vi "Neurosky.vi"() -> ()   [LabVIEW 2011]
uses:
  <vilib>/measure/maspectr.llb/FFT Power Spectrum and PSD for 1 Chan.vi
  Neurosky.lvlib
  <vilib>/measure/NI_MAPro.lvlib
panel:
  out "Mindwave Braiwave Data":T1
  out "FFT Power Spectrum":cluster{"f0":dbl, "df":dbl, "magnitude":dbl[]}(graph)
  out "Mindwave Common Signals\nMobile Data":T2 {"Meditation" scale=0.0..100.0; "Attention" scale=0.0..100.0; "Poor Signal Strength" scale=0.0..255.0}
  out "RAW Wave":waveform(i16)(graph)
  in  "Baud Rate":u16(ring)=10 items=["300", "600", "900", "1200", "2400", "4800", "9600", "19200", "38400", "57600", "115200", "230400"]
  in  "Comm Port":refnum<visa-resource-name>="COM4"
  in  "Start Button":bool
  in  "Stop Button":bool
  # "Visit http://www.cerescontrols.com"
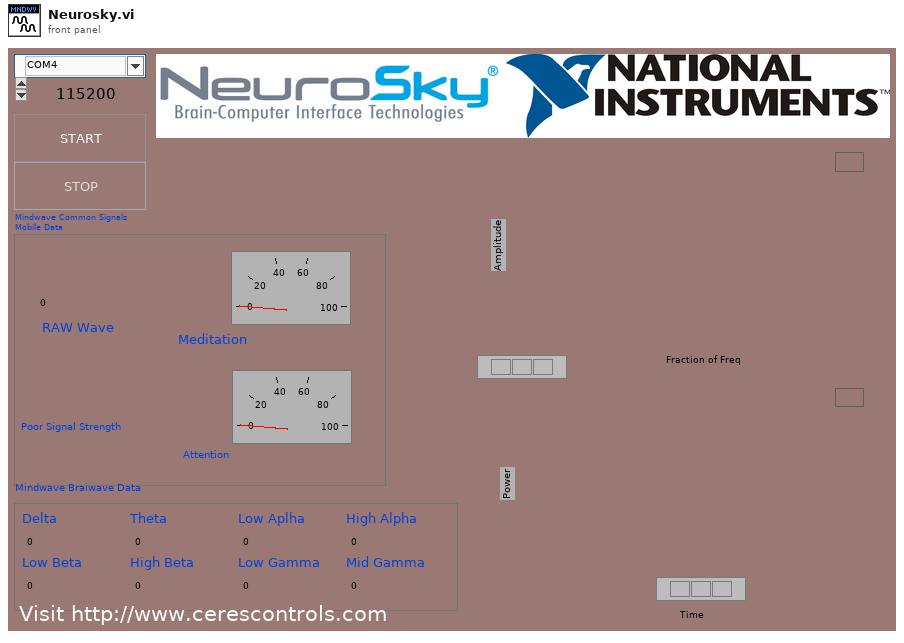
[diagram p1: front panel]
types:
  T1 = cluster{"Delta":sgl, "Theta":sgl, "Low Aplha":sgl, "High Alpha":sgl, "Low Beta":sgl, "High Beta":sgl, "Low Gamma":sgl, "Mid Gamma":sgl}
  T2 = cluster{"RAW Wave":i16, "Poor Signal Strength":u8, "Attention":u16, "Meditation":u8}
  T3 = enum8{"Enabled", "Disabled", "Disabled and Grayed Out"}
  T4 = cluster{"RAW_WAVE":i16, "POOR_QUALITY":u8, "delta":sgl, "theta":sgl, "low alpha":sgl, "high alpha":sgl, "low beta":sgl, "high beta":sgl, "low gamma":sgl, "mid gamma":sgl, "ATTENTION":u8, "MEDITATION":u8}
  T5 = cluster{"delta":sgl, "theta":sgl, "low alpha":sgl, "high alpha":sgl, "low beta":sgl, "high beta":sgl, "low gamma":sgl, "mid gamma":sgl}
  T6 = cluster{"RAW_WAVE":i16, "POOR_QUALITY":u8, "ATTENTION":u8, "MEDITATION":u8}
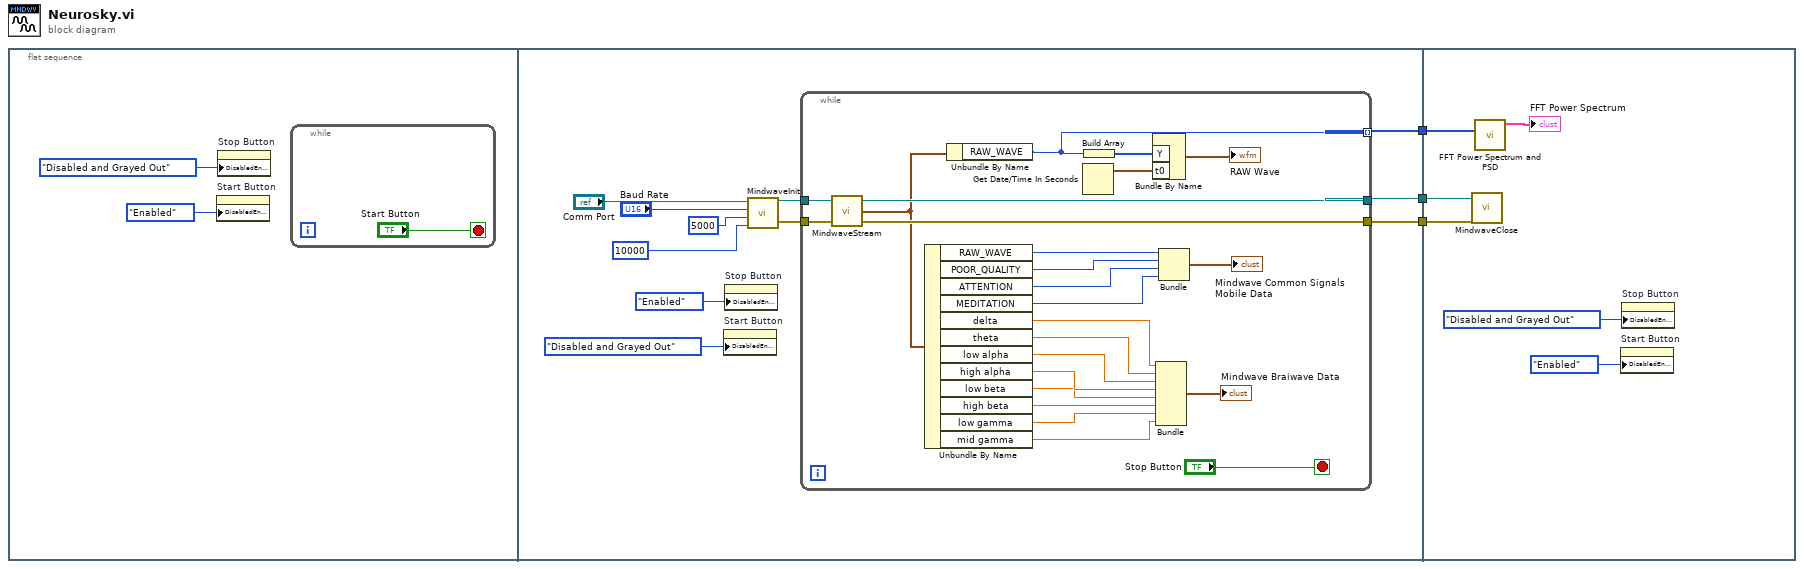
[diagram p0: block diagram]
diagram:
  n1 = flat-sequence {
    tunnel: [w11] -> w3
    tunnel: [w10] -> w2
    tunnel: [w9] -> w1
    tunnel: w3 -> [w47]
    tunnel: w2 -> [w46]
    tunnel: w1 -> [w45]
    frame #0 {
      n2 = property on="Start Button" class="Bool"("DisabledEnum"=T3."Enabled" ("Disabled")) -> ()  [unwired: 2 in, 2 out]
      n3 = property on="Stop Button" class="Bool"("DisabledEnum"=T3."Disabled and Grayed Out" ("Disabled")) -> ()  [unwired: 2 in, 2 out]
      n4 = while {
        stop <- "Start Button" stop-if-true
      }
    }
    frame #1 {
      n5 = property on="Start Button" class="Bool"("DisabledEnum"=T3."Disabled and Grayed Out" ("Disabled")) -> ()  [unwired: 2 in, 2 out]
      n6 = property on="Stop Button" class="Bool"("DisabledEnum"=T3."Enabled" ("Disabled")) -> ()  [unwired: 2 in, 2 out]
      n7 = call <userlib>:"MindwaveInit.vi"("buffer size"=u32 10000, "timeout (10sec)"=u32 5000, "baud rate"="Baud Rate", "COM PORT"="Comm Port") -> ("error out"=w13:errorcluster, "VISA resource name out"=w12:refnum<visa-resource-name>)
      n8 = while {
        tunnel: w13 -> [w22]
        tunnel: w12 -> [w21]
        tunnel: [w37] -> w9 mode=indexing
        tunnel: [w19] -> w11
        tunnel: [w20] -> w10
        stop <- "Stop Button" stop-if-true
        n9 = call <userlib>:"MindwaveStream.vi"("error in (no error) input"=w22, "VISA resource name input"=w21) -> ("error out"=w20:errorcluster, "MindWave"=w18:T4, "VISA resource name out"=w19:refnum<visa-resource-name>)  [unwired: 1 in]
        n10 = Unbundle By Name(w18) -> ("RAW_WAVE"=w36:i16, "POOR_QUALITY"=w33:u8, "ATTENTION"=w34:u8, "MEDITATION"=w35:u8, "delta"=w31:sgl, "theta"=w30:sgl, "low alpha"=w29:sgl, "high alpha"=w28:sgl, "low beta"=w27:sgl, "high beta"=w26:sgl, "low gamma"=w25:sgl, "mid gamma"=w24:sgl)
        n11 = Unbundle By Name(w18) -> ("RAW_WAVE"=w37:i16)
        n12 = Get Date/Time In Seconds() -> (seconds since 1Jan1904=w41:timestamp)
        n13 = Build Array(w37) -> (w40:i16[])
        n14 = Bundle By Name("Y"=w40, "t0"=w41) -> (→"RAW Wave":waveform(i16))  [unwired: 1 in]
        n15 = Bundle("delta"=w31, "theta"=w30, "low alpha"=w29, "high alpha"=w28, "low beta"=w27, "high beta"=w26, "low gamma"=w25, "mid gamma"=w24) -> (→"Mindwave Braiwave Data":T5)  [unwired: 1 in]
        n16 = Bundle("RAW_WAVE"=w36, "POOR_QUALITY"=w33, "ATTENTION"=w34, "MEDITATION"=w35) -> (→"Mindwave Common Signals\nMobile Data":T6)  [unwired: 1 in]
      }
    }
    frame #2 {
      n17 = call <userlib>:"MindwaveClose.vi"("error in (no error)"=w46, "VISA resource name input"=w47) -> ()  [unwired: 1 in]
      n18 = call-poly <vilib>:"FFT Power Spectrum and PSD.vi"("time signal"=w45) -> ("Power Spectrum / PSD"=→"FFT Power Spectrum":cluster{"f0":dbl, "df":dbl, "magnitude":dbl[]})  [unwired: 7 in, 3 out]
      n19 = property on="Start Button" class="Bool"("DisabledEnum"=T3."Enabled" ("Disabled")) -> ()  [unwired: 2 in, 2 out]
      n20 = property on="Stop Button" class="Bool"("DisabledEnum"=T3."Disabled and Grayed Out" ("Disabled")) -> ()  [unwired: 2 in, 2 out]
    }
  }
